vi "Init_graphe.vi"() -> ()   [LabVIEW 2015]
uses:
  <vilib>/Utility/miscctls.llb/LVRowAndColumnTypeDef.ctl
  <vilib>/Utility/file.llb/Read From Spreadsheet File (string).vi
panel:
  in  "Horodatage":timestamp format="%<%I:%M:%S%3u %p>T"
  in  "Bouton Aide":bool
  in  "Quit":bool
  out "horodatage_ok":timestamp format="%<%.3X>T"
  in  "Fichier données":path
  out "Colonne données brutes":string="0"
  out "Ligne données brutes":string="0"
  out "Noms variables":string[](array[string])
  out "Séparateur fichier brute":string
  in  "Valider":bool
  in  "Nouveau format date":bool
  in  "Format d'horodatage":string(combo)="\"%Y-%m-%d %H:%M:%S\""
  in  "Convertir Horodatage":bool
  out "Nb lignes":i32
  in  "Séparateur":u16(ring)=1 items=["", ",", ";", ".", "Tab", "Espace", ":"]
  out "Horodatage_1":timestamp[](array[timestamp]) format="%<%X\n%x>T"
  out "Table":string[][](table)
  out "Donnees":dbl[][](array[numeric])
  in  "Bouton vide 2":bool
  # "Facultatif : \nSélectionner la dernière cellule des noms de variables  en appuyant sur la touche CTRL"
  # "Sélectionner la 1ère cellule\ndes noms de variables"
  # "Sélectionner la 1ère cellule\nd'horodatage"
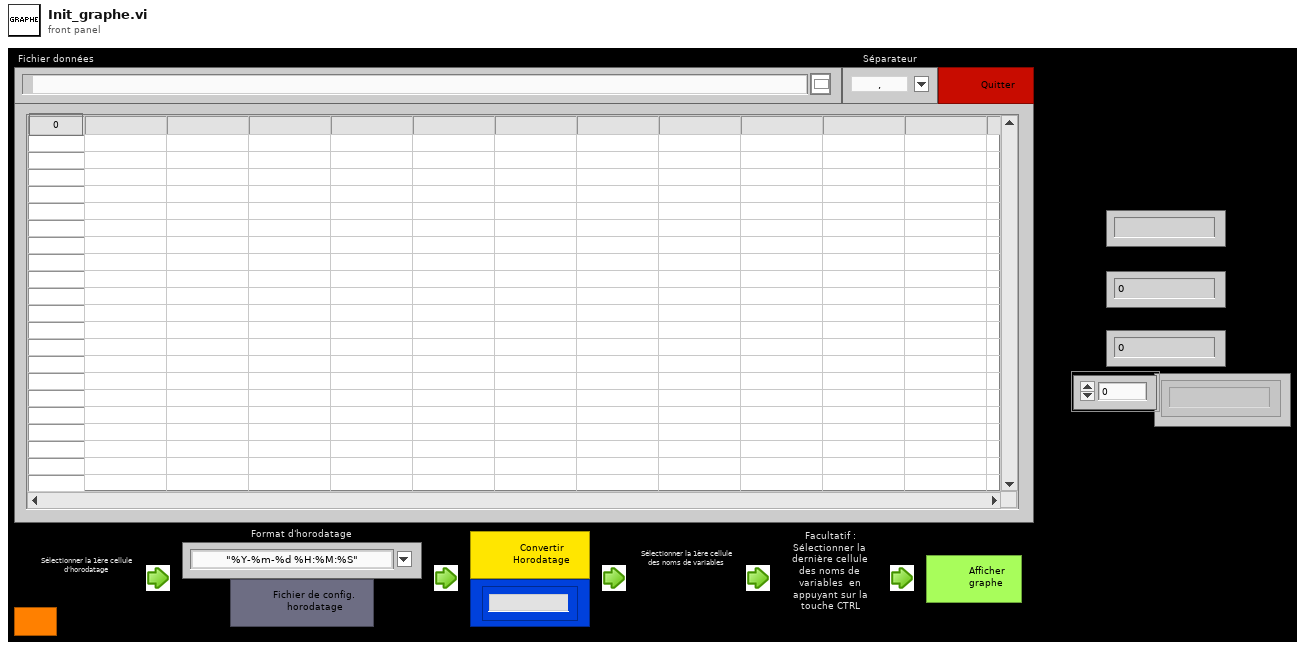
[diagram p1: front panel]
types:
  T1 = typedef "LVRowAndColumnTypeDef.ctl" = cluster{"Row":i32, "Column":i32}
  T2 = typedef "excel Object Reference.ctl" = refnum<k1>
  T3 = enum16{"Left Button", "Center Button", "Right Button", "Window Close"}
  T4 = cluster{"Shift":bool, "Ctrl":bool, "Alt":bool, "Cmd":bool, "Opt":bool}
  T5 = cluster{"Horodatage":timestamp[], "Donnees":dbl[]}[]
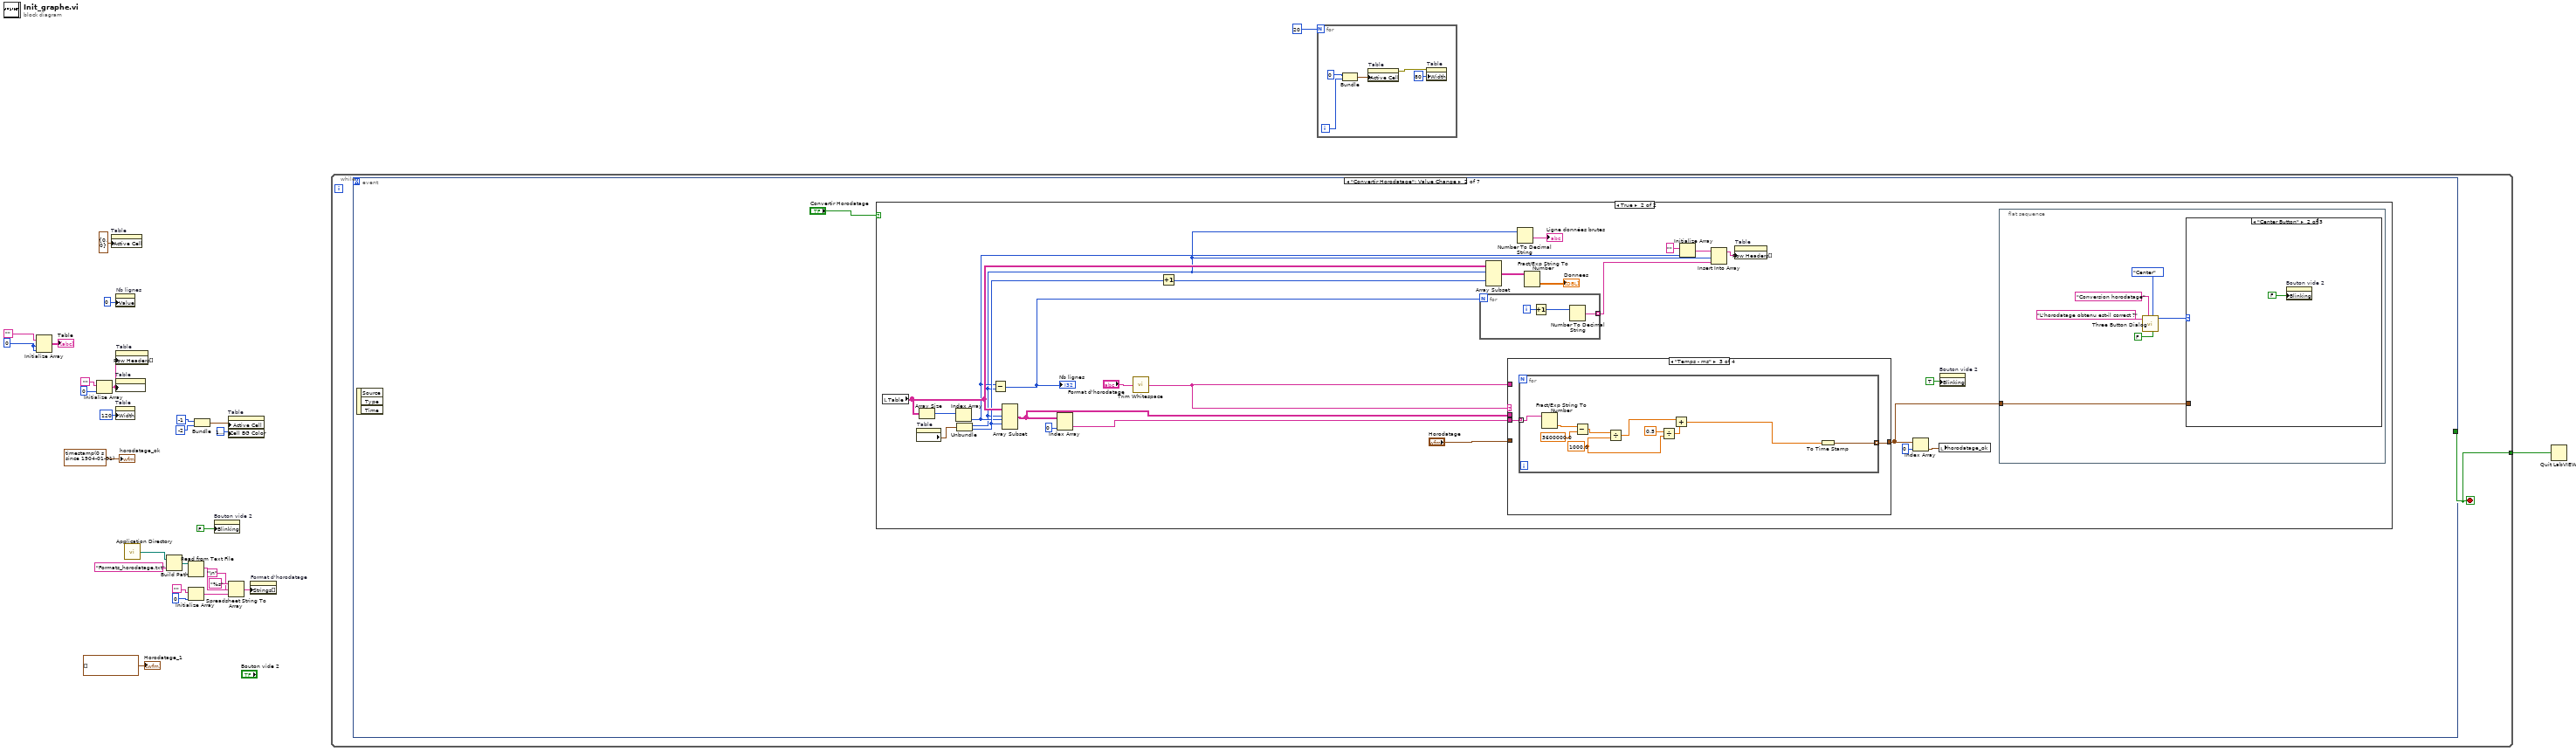
[diagram p0: block diagram]
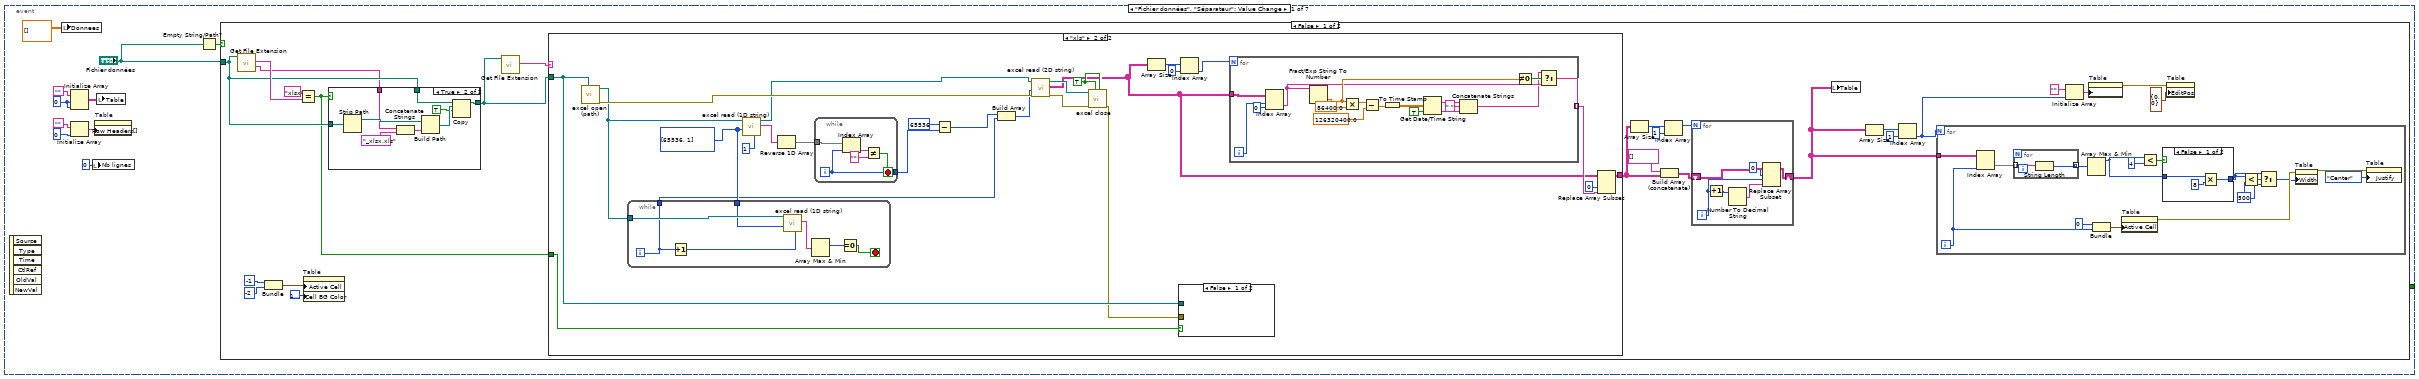
[diagram p2: hidden frame]
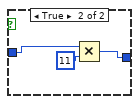
[diagram p4: hidden frame]
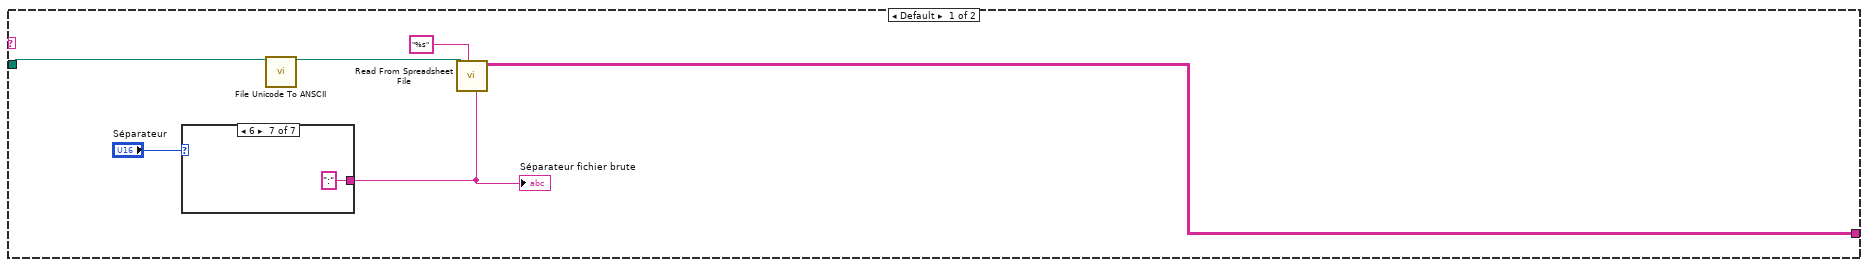
[diagram p5: hidden frame]
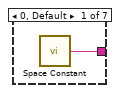
[diagram p6: hidden frame]
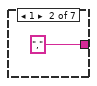
[diagram p7: hidden frame]
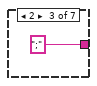
[diagram p8: hidden frame]
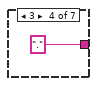
[diagram p9: hidden frame]
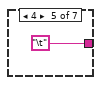
[diagram p10: hidden frame]
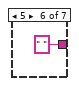
[diagram p11: hidden frame]
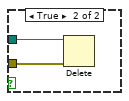
[diagram p12: hidden frame]
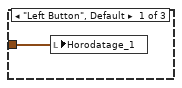
[diagram p15: hidden frame]
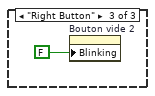
[diagram p16: hidden frame]
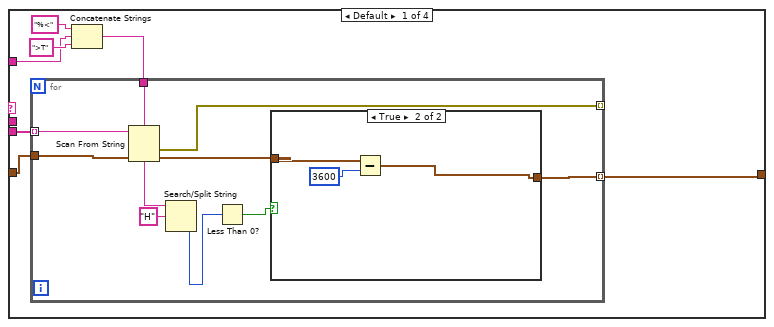
[diagram p17: hidden frame]
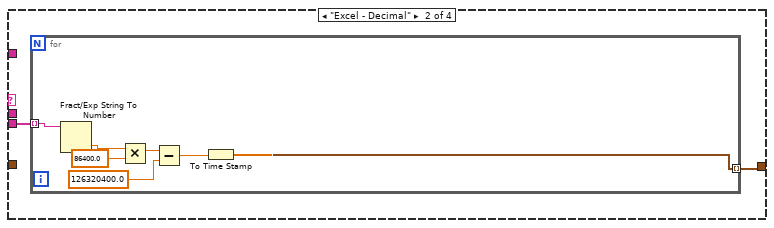
[diagram p19: hidden frame]
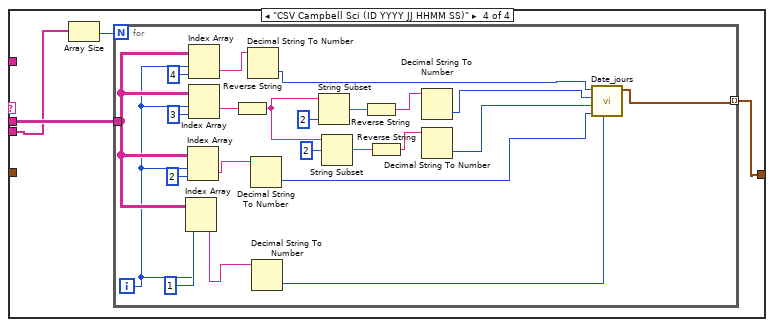
[diagram p20: hidden frame]
diagram:
  w10 = 0 ("taille de la dimension")
  n1 = Initialize Array("", w10, w10) -> (→"Table":string[][])
  n2 = Initialize Array("", 0 ("taille de la dimension")) -> (w17:string[])
  n3 = property on="Table" class="Tbl (strict)"("Active Cell"=T1 {"Row"=0, "Column"=0} ("Cellule active:Cellule active")) -> ()  [unwired: 2 in, 2 out]
  n4 = property on="Table" class="Tbl (strict)"("Column Headers[]"=w17) -> ()  [unwired: 2 in, 2 out]
  n5 = property on="Table" class="Tbl (strict)"("Width"=u32 120 ("Cellule active:Taille de la cellule:Largeur")) -> ()  [unwired: 2 in, 2 out]
  n6 = property on="Nb lignes" class="DigNum (strict)"("Value"=0 ("Nb lignes")) -> ()  [unwired: 2 in, 2 out]
  n7 = property on="Table" class="Tbl (strict)"("Row Headers[]"=w17) -> ()  [unwired: 2 in, 2 out]
  n8 = call <vilib>:"Application Directory.vi"() -> ("Application Directory"=w13:path)
  n9 = Build Path(base path=w13, name or relative path="Formats_horodatage.txt" ("nom ou chemin relatif")) -> (appended path=w21:path)
  n10 = Read from Text File(file (use dialog)=w21) -> (text=w26:string)  [unwired: 3 in, 3 out]
  n11 = Initialize Array("", 0 ("taille de la dimension")) -> (w22:string[])
  n12 = Bundle(-1, -2) -> (w2:cluster{i32, i32})  [unwired: 1 in]
  n13 = property on="Bouton vide 2" class="Bool"("Blinking"=FALSE ("Clignotant")) -> ()  [unwired: 2 in, 2 out]
  n14 = property on="Table" class="Tbl (strict)"("Active Cell"=w2, "Cell BG Color"=u32 16777225) -> ()  [unwired: 2 in, 2 out]
  n15 = Spreadsheet String To Array(delimiter (Tab)="\n", format string="%s" ("chaîne de format"), spreadsheet string=w26, array type (2D Dbl)=w22) -> (array=w18:string[])
  n16 = property on="Format d'horodatage" class="CmbBox"("Strings[]"=w18) -> ()  [unwired: 2 in, 2 out]
  n17 = while {
    tunnel: [w29] -> w7
    stop <- w29 stop-if-true
    n18 = event shown="[1] \"Convertir Horodatage\": Value Change" {
      selector: _ -> [_ _ _ _ _ _ _]
      dyn-events: _ -> [_ _ _ _ _ _ _]
      timeout: _ -> [_ _ _ _ _ _ _]
      tunnel: [_ _ _ _ _ w400 _] -> w29
      event "Fichier données", "Séparateur": Value Change {
        w39 = 0 ("taille de la dimension")
        n19 = event-data() -> ()  [unwired: 1 in, 6 out]
        n20 = local write "Donnees"(dbl[][] [] ("Donnees")) -> ()
        n21 = Initialize Array("", w39, w39) -> (w37:string[][])
        n22 = Initialize Array("", 0 ("taille de la dimension")) -> (w34:string[])
        n23 = local write "Nb lignes"(0 ("Nb lignes")) -> ()
        n24 = property on="Table" class="Tbl (strict)"("Row Headers[]"=w34) -> ()  [unwired: 2 in, 2 out]
        n25 = local write "Table"(w37) -> ()
        n26 = Empty String/Path?(string/path="Fichier données") -> (empty?=w31:bool)
        n27 = case shown="False" w31 {
          tunnel: "Fichier données" -> [w44 _]
          frame False {
            n28 = call <vilib>:"Get File Extension.vi"("file"=w44) -> ("filename without extension"=w43:string, "lowercase file extension"=w46:string)  [unwired: 6 in, 3 out]
            n29 = Bundle(-1, -2) -> (w57:cluster{i32, i32})  [unwired: 1 in]
            n30 = Equal?(x="xlsx", y=w46) -> (x = y?=w40:bool)
            n31 = property on="Table" class="Tbl (strict)"("Active Cell"=w57, "Cell BG Color"=u32 16777225) -> ()  [unwired: 2 in, 2 out]
            n32 = case shown="True" w40 {
              tunnel: w44 -> [w65 w74]
              tunnel: [w65 w73] -> w42
              tunnel: w44 -> [_ w71]
              tunnel: w43 -> [_ w68]
              frame False {
              }
              frame True {
                n33 = Strip Path(path=w71) -> (stripped path=w72:path)  [unwired: 1 out]
                n34 = Concatenate Strings(w68, "_xlsx.xls" ("chaîne")) -> (w69:string)
                n35 = Build Path(base path=w72, name or relative path=w69) -> (appended path=w70:path)
                n36 = Copy(9:TRUE ("écraser (F)"), 10:w70, 11:w74) -> (3:w73:path)  [unwired: 2 in, 2 out]
              }
            }
            n37 = call <vilib>:"Get File Extension.vi"("file"=w42) -> ("lowercase file extension"=w41:string)  [unwired: 6 in, 4 out]
            n38 = case shown="\"xls\"" w41 {
              tunnel: w42 -> [w106 w127]
              tunnel: [w108 w128] -> w50
              tunnel: w40 -> [_ w125]
              frame Default {
                n39 = case shown="6" "Séparateur" {
                  tunnel: [w111 "," ";" "." "\t" " " ("String") ":" ("String")] -> w107
                  frame 0, Default {
                    n40 = call <vilib>:"Space Constant.vi"() -> ("String"=w111:string)
                  }
                  frame 1 {
                  }
                  frame 2 {
                  }
                  frame 3 {
                  }
                  frame 4 {
                  }
                  frame 5 {
                  }
                  frame 6 {
                  }
                }
                "Séparateur fichier brute" <- w107
                n41 = call "File Unicode To ANSCII.vi"("file in"=w106) -> ("file out"=w105:path)  [unwired: 18 in]
                n42 = call-poly <vilib>:"Read From Spreadsheet File.vi"("delimiter (\\t)"=w107, "format (%s)"="%s", "file path (dialog if empty)"=w105) -> ("all rows"=w108:string[][])  [unwired: 4 in, 4 out]
              }
              frame "xls" {
                w122 = i32[] [65536, 1] ("array size\n  - #rows\n  - #columns")
                w139 = TRUE ("Override closing behavior")
                n43 = call "excel open (path).vi"("workbook path"=w127) -> ("error out"=w140:errorcluster, "reference"=w124:T2)  [unwired: 9 in]
                n44 = while {
                  tunnel: w124 -> [w148]
                  tunnel: w122 -> [w146]
                  tunnel: [w143] -> w121
                  i -> [w143]
                  stop <- w149 stop-if-true
                  n45 = Increment(x=w143) -> (x+1=w147:i32)
                  n46 = call "excel read (1D string).vi"("Column"=w147, "array size\n  - #rows\n  - #columns"=w146, "reference"=w148) -> ("1D String Array"=w145:string[])  [unwired: 6 in, 2 out]
                  n47 = Array Max & Min(array=w145) -> (max index (indices)=w144:i32)  [unwired: 3 out]
                  n48 = Equal To 0?(x=w144) -> (x = 0?=w149:bool)
                }
                n49 = call "excel read (1D string).vi"("Column"=u32 1, "array size\n  - #rows\n  - #columns"=w122, "reference"=w124) -> ("1D String Array"=w138:string[], "duplicate reference"=w118:T2)  [unwired: 6 in, 1 out]
                n50 = Reverse 1D Array(array=w138) -> (reversed array=w137:string[])
                n51 = while {
                  tunnel: w137 -> [w173]
                  tunnel: [w169] -> w136
                  i -> [w169]
                  stop <- w170 stop-if-true
                  n52 = Index Array(array=w173, index=w169) -> (element=w172:string)
                  n53 = Not Equal?(x=w172, y="") -> (x != y?=w170:bool)
                }
                n54 = Subtract(x=65536, y=w136) -> (x-y=w120:i32)
                n55 = Build Array(w120, w121) -> (w123:i32[])
                n56 = call "excel read (2D string).vi"("error in (no error)"=w140, "array size\n  - #rows\n  - #columns"=w123, "reference"=w118) -> ("error out"=w141:errorcluster, "2D String Array"=w129:string[][], "duplicate reference"=w142:T2)  [unwired: 6 in]
                n57 = call "excel close.vi"("Close"=w139, "Override closing behavior"=w139, "error in (no error)"=w141, "reference"=w142) -> ("error out"=w126:errorcluster)  [unwired: 7 in]
                n58 = Array Size(array=w129) -> (size(s)=w131:i32[])
                n59 = case shown="False" w125 {
                  tunnel: w127 -> [_ w151]
                  tunnel: w126 -> [_ w150]
                  frame False {
                  }
                  frame True {
                    n60 = Delete(path (use dialog)=w151, error in=w150) -> ()  [unwired: 3 in, 3 out]
                  }
                }
                n61 = Index Array(array=w131, index=0 ("indice")) -> (element=w132:i32)
                n62 = for {
                  N: w132 -> [_]
                  tunnel: w129 -> [w168]
                  tunnel: [w153] -> w134 mode=indexing
                  i -> [w167]
                  n63 = Index Array(array=w168, index (row)=w167, index (col)=0 ("indice désactivé (col)")) -> (element=w154:string)
                  n64 = Fract/Exp String To Number(string=w154) -> (number=w155:dbl)  [unwired: 3 in, 1 out]
                  n65 = Multiply(x=w155, y=86400.0) -> (x*y=w164:dbl)
                  n66 = Subtract(x=w164, y=126320400.0) -> (x-y=w162:dbl)
                  n67 = To Time Stamp(1:w162) -> (0:w161:timestamp)
                  n68 = Get Date/Time String(seconds (now)=w161, want seconds? (F)=TRUE ("secondes ? (F)")) -> (date string=w159:string, time string=w157:string)  [unwired: 1 in]
                  n69 = Concatenate Strings(w159, " " ("chaîne"), w157) -> (w152:string)
                  n70 = Not Equal To 0?(x=w155) -> (x != 0?=w156:bool)
                  n71 = Select(t=w152, s=w156, f=w154) -> (s? t:f=w153:string)
                }
                n72 = Replace Array Subset(array=w129, new element=w134, index (col)=0 ("indice désactivé (col)")) -> (w128:string[][])  [unwired: 1 in]
              }
            }
            n73 = Array Size(array=w50) -> (size(s)=w52:i32[])
            n74 = Build Array (concatenate)(string[] [] ("élément"), w50) -> (w48:string[][])
            n75 = Index Array(array=w52, index=1 ("indice")) -> (element=w51:i32)
            n76 = for {
              N: w51 -> [_]
              shift-right: [w80] -> w54
              shift-left: w48 -> [w79]
              i -> [w76]
              n77 = Increment(x=w76) -> (x+1=w78:i32)
              n78 = Number To Decimal String(number=w78) -> (decimal integer string=w75:string)  [unwired: 1 in]
              n79 = Replace Array Subset(array=w79, new element=w75, index (row)=0 ("indice désactivé (ligne)"), index (col)=w76) -> (w80:string[][])
            }
            n80 = local write "Table"(w54) -> ()
            n81 = Array Size(array=w54) -> (size(s)=w60:i32[])
            n82 = Index Array(array=w60, index=1 ("indice")) -> (element=w47:i32)
            n83 = for {
              N: w47 -> [_]
              tunnel: w54 -> [w96]
              i -> [w91]
              w82 = 500 ("cas faux")
              n84 = Index Array(array=w96, index (col)=w91) -> (element=w95:string[])  [unwired: 1 in]
              n85 = for {
                tunnel: w95 -> [w104] mode=indexing
                tunnel: [w103] -> w94 mode=indexing
                n86 = String Length(string=w104) -> (length=w103:i32)
              }
              n87 = Array Max & Min(array=w94) -> (max value=w86:i32)  [unwired: 3 out]
              n88 = Bundle(0, w91) -> (w93:cluster{i32, i32})  [unwired: 1 in]
              n89 = property on="Table" class="Tbl (strict)"("Active Cell"=w93) -> (error out=w92:errorcluster)  [unwired: 2 in, 1 out]
              n90 = Less?(x=w86, y=4) -> (x < y?=w87:bool)
              n91 = case shown="False" w87 {
                tunnel: [w99 w100] -> w81
                tunnel: w86 -> [w97 w101]
                frame False {
                  n92 = Multiply(x=w97, y=8) -> (x*y=w99:i32)
                }
                frame True {
                  n93 = Multiply(x=w101, y=11) -> (x*y=w100:i32)
                }
              }
              n94 = Less?(x=w81, y=w82) -> (x < y?=w83:bool)
              n95 = Select(t=w81, s=w83, f=w82) -> (s? t:f=w84:i32)
              n96 = property on="Table" class="Tbl (strict)"(error in=w92, "Width"=w84) -> (error out=w89:errorcluster)  [unwired: 1 in, 1 out]
              n97 = property on="Table" class="Tbl (strict)"(error in=w89, "Justify"=enum16{"Left", "Center", "Right"}."Center" ("Cellule active:Justification de la cellule")) -> ()  [unwired: 1 in, 2 out]
            }
            n98 = Initialize Array("", w47) -> (w63:string[])
            n99 = property on="Table" class="Tbl (strict)"("Column Headers[]"=w63) -> (error out=w61:errorcluster)  [unwired: 2 in, 1 out]
            n100 = property on="Table" class="Tbl (strict)"(error in=w61, "EditPos"=T1 {"Row"=0, "Column"=0} ("Cellule active:Cellule active")) -> ()  [unwired: 1 in, 2 out]
          }
          frame True {
          }
        }
      }
      event "Convertir Horodatage": Value Change {
        n101 = event-data() -> ()  [unwired: 1 in, 3 out]
        n102 = case shown="True" "Convertir Horodatage" {
          frame False {
          }
          frame True {
            n103 = local read "Table"() -> (w194:string[][])
            n104 = property on="Table" class="Tbl (strict)"() -> ("Selection Start"=w197:T1)  [unwired: 2 in, 2 out]
            n105 = Array Size(array=w194) -> (size(s)=w195:i32[])
            n106 = Index Array(array=w195) -> (element=w189:i32)  [unwired: 1 in]
            n107 = Unbundle(w197) -> ("Row"=w185:i32, "Column"=w190:i32)
            n108 = Subtract(x=w189, y=w185) -> (x-y=w180:i32)
            "Nb lignes" <- w180
            n109 = Array Subset(array=w194, index (row)=w185, length (row)=w189, index (col)=w190) -> (w182:string[][])  [unwired: 1 in]
            n110 = Index Array(array=w182, index (col)=0 ("indice (ligne)")) -> (element=w187:string[])  [unwired: 1 in]
            n111 = call <vilib>:"Trim Whitespace.vi"("string"="Format d'horodatage") -> ("trimmed string"=w176:string)  [unwired: 1 in]
            n112 = Increment(x=w190) -> (x+1=w196:i32)
            n113 = for {
              N: w180 -> [_]
              tunnel: [w278] -> w191 mode=indexing
              i -> [w279]
              n114 = Increment(x=w279) -> (x+1=w277:i32)
              n115 = Number To Decimal String(number=w277) -> (decimal integer string=w278:string)  [unwired: 1 in]
            }
            n116 = Array Subset(array=w194, index (row)=w185, index (col)=w196) -> (w198:string[][])  [unwired: 2 in]
            n117 = case shown="\"Temps - ms\"" w176 {
              tunnel: "Horodatage" -> [w215 _ _ _]
              tunnel: w187 -> [w212 w230 w239 w250]
              tunnel: [w211 w229 w238 w252] -> w179
              tunnel: w176 -> [w209 _ _ _]
              tunnel: w182 -> [_ _ _ w253]
              frame Default {
                n118 = Concatenate Strings("%<", w209, ">T") -> (w210:string)
                n119 = for {
                  tunnel: [w219] -> w211 mode=indexing
                  tunnel: w215 -> [w224]
                  tunnel: w210 -> [w222]
                  tunnel: w212 -> [w223] mode=indexing
                  tunnel: [w216] -> _ mode=indexing
                  n120 = Scan From String(format string=w222, input string=w223, default 1=w224) -> (error out=w216:errorcluster, output 1=w220:timestamp)  [unwired: 2 in, 2 out]
                  n121 = Search/Split String(string=w222, search string/char (-)="H" ("chaîne/car. recherché (-)")) -> (offset of match=w218:i32)  [unwired: 1 in, 2 out]
                  n122 = Less Than 0?(x=w218) -> (x < 0?=w217:bool)
                  n123 = case shown="True" w217 {
                    tunnel: w220 -> [w225 w228]
                    tunnel: [w225 w226] -> w219
                    frame False {
                    }
                    frame True {
                      n124 = Subtract(x=w228, y=3600) -> (x-y=w226:timestamp)
                    }
                  }
                }
              }
              frame "Excel - Decimal" {
                n125 = for {
                  tunnel: [w231] -> w229 mode=indexing
                  tunnel: w230 -> [w237] mode=indexing
                  n126 = Fract/Exp String To Number(string=w237) -> (number=w236:dbl)  [unwired: 3 in, 1 out]
                  n127 = Multiply(x=w236, y=86400.0) -> (x*y=w234:dbl)
                  n128 = Subtract(x=w234, y=126320400.0) -> (x-y=w232:dbl)
                  n129 = To Time Stamp(1:w232) -> (0:w231:timestamp)
                }
              }
              frame "Temps - ms" {
                n130 = for {
                  tunnel: [w248] -> w238 mode=indexing
                  tunnel: w239 -> [w249] mode=indexing
                  w241 = 1000.0 ("y")
                  n131 = Fract/Exp String To Number(string=w249) -> (number=w246:dbl)  [unwired: 3 in, 1 out]
                  n132 = Subtract(x=w246, y=3600000.0) -> (x-y=w245:dbl)
                  n133 = Divide(x=w245, y=w241) -> (x/y=w244:dbl)
                  n134 = Divide(x=0.5, y=w241) -> (x/y=w243:dbl)
                  n135 = Add(x=w244, y=w243) -> (x+y=w240:dbl)
                  n136 = To Time Stamp(1:w240) -> (0:w248:timestamp)
                }
              }
              frame "CSV Campbell Sci (ID YYYY JJ HHMM SS)" {
                n137 = Array Size(array=w250) -> (size(s)=w251:i32)
                n138 = for {
                  N: w251 -> [_]
                  tunnel: w253 -> [w263]
                  tunnel: [w254] -> w252 mode=indexing
                  i -> [w262]
                  n139 = Index Array(array=w263, index (row)=w262, index (col)=1 ("indice désactivé (col)")) -> (element=w260:string)
                  n140 = Index Array(array=w263, index (row)=w262, index (col)=2 ("indice désactivé (col)")) -> (element=w261:string)
                  n141 = Index Array(array=w263, index (row)=w262, index (col)=4 ("indice désactivé (col)")) -> (element=w275:string)
                  n142 = Index Array(array=w263, index (row)=w262, index (col)=3 ("indice désactivé (col)")) -> (element=w273:string)
                  n143 = Reverse String(1:w273) -> (0:w269:string)
                  n144 = Decimal String To Number(string=w275) -> (number=w259:i32)  [unwired: 2 in, 1 out]
                  n145 = Decimal String To Number(string=w261) -> (number=w256:i32)  [unwired: 2 in, 1 out]
                  n146 = Decimal String To Number(string=w260) -> (number=w255:i32)  [unwired: 2 in, 1 out]
                  n147 = String Subset(string=w269, length (rest)=2 ("longueur (reste)")) -> (substring=w271:string)  [unwired: 1 in]
                  n148 = String Subset(string=w269, offset (0)=2) -> (substring=w267:string)  [unwired: 1 in]
                  n149 = Reverse String(1:w271) -> (0:w270:string)
                  n150 = Reverse String(1:w267) -> (0:w266:string)
                  n151 = Decimal String To Number(string=w270) -> (number=w258:i32)  [unwired: 2 in, 1 out]
                  n152 = Decimal String To Number(string=w266) -> (number=w257:i32)  [unwired: 2 in, 1 out]
                  n153 = call "Date_jours.vi"("year"=w255, "jours n"=w256, "hour"=w257, "minute"=w258, "second"=w259) -> ("horodatage"=w254:timestamp)  [unwired: 6 in]
                }
              }
            }
            n154 = Number To Decimal String(number=w185) -> (decimal integer string=→"Ligne données brutes":string)  [unwired: 1 in]
            n155 = Fract/Exp String To Number(string=w198) -> (number=→"Donnees":dbl[][])  [unwired: 3 in, 1 out]
            n156 = Initialize Array("", w189) -> (w192:string[])
            n157 = Insert Into Array(array=w192, index=w185, new element=w191) -> (w181:string[])
            n158 = property on="Table" class="Tbl (strict)"("Row Headers[]"=w181) -> ()  [unwired: 2 in, 2 out]
            n159 = Index Array(array=w179, index=0 ("indice")) -> (element=w178:timestamp)
            n160 = local write "horodatage_ok"(w178) -> ()
            n161 = property on="Bouton vide 2" class="Bool"("Blinking"=TRUE ("Clignotant")) -> ()  [unwired: 2 in, 2 out]
            n162 = flat-sequence {
              tunnel: w179 -> [w200]
              frame #0 {
                n163 = call <vilib>:"Three Button Dialog.vi"("Allow user to close window? (TRUE)"=FALSE, "Justify Message (Left)"=enum16{"Left", "Center", "Right"}."Center", "Window Title (\"\")"="Conversion horodatage" ("error source (\" \")"), "message"="L'horodatage obtenu est-il correct ?" ("error source (\" \")")) -> ("Which Button?"=w203:T3)  [unwired: 7 in]
                n164 = case shown="\"Center Button\"" w203 {
                  tunnel: w200 -> [w206 _ _]
                  frame "Left Button", Default {
                    n165 = local write "Horodatage_1"(w206) -> ()
                  }
                  frame "Center Button" {
                    n166 = property on="Bouton vide 2" class="Bool"("Blinking"=FALSE ("Clignotant")) -> ()  [unwired: 2 in, 2 out]
                  }
                  frame "Right Button" {
                    n167 = property on="Bouton vide 2" class="Bool"("Blinking"=FALSE ("Clignotant")) -> ()  [unwired: 2 in, 2 out]
                  }
                }
              }
            }
          }
        }
      }
      event "Nouveau format date": Value Change {
        n168 = event-data() -> ()  [unwired: 1 in, 6 out]
        n169 = call <vilib>:"Application Directory.vi"() -> ("Application Directory"=w280:path)
        n170 = Build Path(base path=w280, name or relative path="Formats_horodatage.txt" ("nom ou chemin relatif")) -> (appended path=w282:path)
        n171 = Path To String(path=w282) -> (string=w283:string)
        n172 = Concatenate Strings("cmd /c NOTEPAD " ("command line"), w283) -> (w285:string)
        n173 = flat-sequence {
          tunnel: w285 -> [w289]
          tunnel: w282 -> [w287]
          tunnel: [w287] -> w281
          tunnel: w281 -> [w290]
          frame #0 {
            n174 = call <vilib>:"System Exec.vi"("run minimized? (F)"=TRUE, "command line"=w289) -> ()  [unwired: 6 in, 4 out]
          }
          frame #1 {
            n175 = Read from Text File(file (use dialog)=w290) -> (text=w291:string)  [unwired: 3 in, 3 out]
            n176 = Initialize Array("", 0 ("taille de la dimension")) -> (w295:string[])
            n177 = Spreadsheet String To Array(delimiter (Tab)="\n", format string="%s" ("chaîne de format"), spreadsheet string=w291, array type (2D Dbl)=w295) -> (array=w297:string[])
            n178 = property on="Format d'horodatage" class="CmbBox"("Strings[]"=w297) -> ()  [unwired: 2 in, 2 out]
          }
        }
      }
      event "Table": Mouse Down {
        n179 = event-data() -> ("PlatMods"=w305:T4)  [unwired: 1 in, 7 out]
        n180 = local read "Horodatage_1"() -> (w304:timestamp[])
        n181 = property on="Table" class="Tbl (strict)"() -> ("Selection Start"=w300:T1)  [unwired: 2 in, 2 out]
        n182 = Array Size(array=w304) -> (size(s)=w303:i32)
        n183 = Equal To 0?(x=w303) -> (x = 0?=w301:bool)
        n184 = Unbundle(w300) -> ("Column"=w299:i32)  [unwired: 1 out]
        n185 = Equal To 0?(x=w299) -> (x = 0?=w298:bool)
        n186 = Or(x=w298, y=w301) -> (x .or. y?=w302:bool)
        n187 = case shown="False" w302 {
          tunnel: w305 -> [w312 _]
          frame False {
            n188 = Unbundle(w312) -> ("Ctrl"=w311:bool)  [unwired: 4 out]
            n189 = case shown="True" w311 {
              tunnel: [w336 w355] -> w308
              tunnel: [w334 w355] -> w307
              frame False {
                n190 = local read "Table"() -> (w333:string[][])
                n191 = property on="Table" class="Tbl (strict)"() -> ("Selection Start"=w335:T1)  [unwired: 2 in, 2 out]
                n192 = Array Size(array=w333) -> (size(s)=w346:i32[])
                n193 = Unbundle(w335) -> ("Row"=w337:i32, "Column"=w339:i32)
                n194 = Index Array(array=w346, index=1 ("indice")) -> (element=w340:i32)
                n195 = Subtract(x=w340, y=w339) -> (x-y=w344:i32)
                n196 = Number To Decimal String(number=w339) -> (decimal integer string=→"Colonne données brutes":string)  [unwired: 1 in]
                n197 = Array Subset(array=w333, index (row)=w337, length (row)=1 ("longueur"), index (col)=w339, length (col)=w344) -> (w347:string[][])
                n198 = Index Array(array=w347, index (row)=0 ("indice (ligne)")) -> (element=w336:string[])  [unwired: 1 in]
                n199 = Initialize Array("", w340) -> (w342:string[])
                n200 = Replace Array Subset(array=w342, new element=w336, index=w339) -> (w334:string[])
                n201 = property on="Table" class="Tbl (strict)"("Column Headers[]"=w334) -> ()  [unwired: 2 in, 2 out]
              }
              frame True {
                n202 = Bundle(-1, -2) -> (w352:cluster{i32, i32})  [unwired: 1 in]
                n203 = property on="Table" class="Tbl (strict)"("Active Cell"=w352, "Cell BG Color"=u32 16777225) -> ()  [unwired: 2 in, 2 out]
                n204 = property on="Table" class="Tbl (strict)"() -> ("Column Headers[]"=w354:string[], "Selection Start"=w349:T1)  [unwired: 2 in, 2 out]
                n205 = Unbundle(w349) -> ("Column"=w356:i32)  [unwired: 1 out]
                n206 = Increment(x=w356) -> (x+1=w358:i32)
                n207 = Array Subset(array=w354, index=0 ("indice"), length=w358) -> (w355:string[])
                n208 = property on="Table" class="Tbl (strict)"("Column Headers[]"=w355) -> ()  [unwired: 2 in, 2 out]
              }
            }
            n209 = for {
              tunnel: w308 -> [w321] mode=indexing
              shift-right: [w323] -> w310
              shift-left: string[] [] -> [w324]
              n210 = Search and Replace String(replace all?=TRUE ("tout remplacer ? (F)"), input string=w321, search string="\"" ("chaîne recherchée"), replace string="" ("chaîne de remplacement (\"\")")) -> (result string=w322:string)  [unwired: 4 in, 3 out]
              n211 = Empty String/Path?(string/path=w322) -> (empty?=w325:bool)
              n212 = case shown="True" w325 {
                tunnel: w324 -> [w331 w332]
                tunnel: [w329 w332] -> w323
                tunnel: w322 -> [w330 _]
                frame False {
                  n213 = Build Array (concatenate)(w331, w330) -> (w329:string[])
                }
                frame True {
                }
              }
            }
            "Noms variables" <- w310
            n214 = for {
              tunnel: w307 -> [w320] mode=indexing
              i -> [w318]
              n215 = Empty String/Path?(string/path=w320) -> (empty?=w316:bool)
              n216 = Bundle(-1, w318) -> (w317:cluster{i32, i32})  [unwired: 1 in]
              n217 = Select(t=u32 16777225, s=w316, f=u32 10473471) -> (s? t:f=w313:u32)
              n218 = property on="Table" class="Tbl (strict)"("Active Cell"=w317, "Cell BG Color"=w313) -> ()  [unwired: 2 in, 2 out]
            }
          }
          frame True {
          }
        }
        n219 = property on="Table" class="Tbl (strict)"("Selection Size"=T1 {"Row"=1, "Column"=1} ("Taille de sélection")) -> ()  [unwired: 2 in, 2 out]
      }
      event "Valider": Value Change {
        n220 = event-data() -> ()  [unwired: 1 in, 6 out]
        n221 = property on="Table" class="Tbl (strict)"() -> ("Column Headers[]"=w364:string[])  [unwired: 2 in, 2 out]
        n222 = local read "Horodatage_1"() -> (w369:timestamp[])
        n223 = Sort 1D Array(array=w364) -> (sorted array=w363:string[])
        n224 = Array Size(array=w369) -> (size(s)=w368:i32)
        n225 = Reverse 1D Array(array=w363) -> (reversed array=w359:string[])
        n226 = Not Equal To 0?(x=w368) -> (x != 0?=w365:bool)
        n227 = Index Array(array=w359) -> (element=w362:string)  [unwired: 1 in]
        n228 = property on="Table" class="Tbl (strict)"("Selection Size"=T1 {"Row"=1, "Column"=1} ("Taille de sélection")) -> ()  [unwired: 2 in, 2 out]
        n229 = Empty String/Path?(string/path=w362) -> (empty?=w361:bool)
        n230 = Not(x=w361) -> (.not. x?=w360:bool)
        n231 = And(x=w360, y=w365) -> (x .and. y?=w366:bool)
        n232 = case shown="True" w366 {
          tunnel: "Valider" -> [_ w377]
          tunnel: w369 -> [_ w376]
          frame False {
            w373 = "" ("Left Button Text (\"Yes\")")
            n233 = call <vilib>:"Three Button Dialog.vi"("Justify Message (Left)"=enum16{"Left", "Center", "Right"}."Center", "Window Title (\"\")"="Problème affichage graphe" ("Window Title (\"\")"), "Right Button Text (\"Cancel\")"=w373, "Center Button Text (\"No\")"="Ok" ("Center Button Text (\"No\")"), "Left Button Text (\"Yes\")"=w373, "message"="Veuillez convertir les dates - heures\net sélectionner au moins une variable\npour afficher le graphe") -> ()  [unwired: 5 in, 1 out]
          }
          frame True {
            n234 = case shown="True" w377 {
              tunnel: w376 -> [_ w383]
              frame False {
              }
              frame True {
                n235 = local read "Table"() -> (w393:string[][])
                n236 = property on="Table" class="Tbl (strict)"() -> ("Selection Start"=w379:T1)  [unwired: 2 in, 2 out]
                n237 = Array Size(array=w393) -> (size(s)=w392:i32[])
                n238 = Unbundle(w379) -> ("Row"=w388:i32, "Column"=w387:i32)
                n239 = Index Array(array=w392, index=1 ("indice")) -> (element=w384:i32)
                n240 = Subtract(x=w384, y=w387) -> (x-y=w390:i32)
                n241 = Array Subset(array=w393, index (row)=w388, length (row)=1 ("longueur"), index (col)=w387, length (col)=w390) -> (w395:string[][])
                n242 = Index Array(array=w395, index (row)=0 ("indice (ligne)")) -> (element=w382:string[])  [unwired: 1 in]
                n243 = Initialize Array("", w384) -> (w386:string[])
                n244 = Replace Array Subset(array=w386, new element=w382, index=w387) -> ()  [unwired: 1 out]
                n245 = local read "Donnees"() -> (w394:dbl[][])
                n246 = property on="Table" class="Tbl (strict)"() -> ("Column Headers[]"=w378:string[])  [unwired: 2 in, 2 out]
                n247 = call "MAJ_Graphe.vi"("Horodatage"=w383, "Donnees"=w394, "Entetes colonnes"=w378) -> ("Graphe"=w381:T5, "Paramètres à afficher"=w380:string[])  [unwired: 5 in]
                n248 = flat-sequence {
                  tunnel: w381 -> [w398]
                  tunnel: w380 -> [w397]
                  frame #0 {
                    n249 = call "Graphe_XY.vi"("Graphe"=w398, "Tableau de chaînes"=w397) -> ()  [unwired: 9 in]
                  }
                  frame #1 {
                    n250 = property on="Table" class="Tbl (strict)"("Active Cell"=T1 {"Row"=0, "Column"=0} ("Cellule active:Cellule active")) -> ()  [unwired: 2 in, 2 out]
                  }
                }
              }
            }
          }
        }
      }
      event "Quit": Value Change {
        n251 = event-data() -> ("NewVal"=w400:bool)  [unwired: 1 in, 5 out]
      }
      event "Bouton Aide": Value Change {
        n252 = event-data() -> ()  [unwired: 1 in, 6 out]
        n253 = call <vilib>:"Application Directory.vi"() -> ("Application Directory"=w402:path)
        n254 = Build Path(base path=w402, name or relative path="Logiciel GRAPHE_Instruction.pdf" ("standard input")) -> (appended path=w401:path)
        n255 = call "Open PDF.vi"("Path"=w401) -> ()  [unwired: 5 in, 2 out]
      }
    }
  }
  n256 = for {
    N: 20 -> [_]
    i -> [w406]
    n257 = Bundle(0, w406) -> (w407:cluster{i32, i32})  [unwired: 1 in]
    n258 = property on="Table" class="Tbl (strict)"("Active Cell"=w407) -> (error out=w404:errorcluster)  [unwired: 2 in, 1 out]
    n259 = property on="Table" class="Tbl (strict)"(error in=w404, "Width"=u32 80 ("Cellule active:Taille de la cellule:Largeur")) -> ()  [unwired: 1 in, 2 out]
  }
  n260 = Quit LabVIEW(quit? (T)=w7) -> ()
  "Horodatage_1" <- timestamp[] [] ("Horodatage")
  "horodatage_ok" <- timestamp(0 s since 1904-01-01)
